vi "prepareToAck.vi"(8 "error in (no error)":errorcluster, 9 "cmdStatus":string(combo)="ack", 10 "cmd":string, 11 "TcpServer in":refnum<class "TcpServer.lvclass">) -> (0 "error out":errorcluster, 2 "JSON string":string, 3 "TcpServer out":refnum<class "TcpServer.lvclass">)   [LabVIEW 2018, in "TcpServer.lvclass"]
doc: "Prepare the command received to do the acknowledgement to the client."
uses:
  TcpServer.lvclass
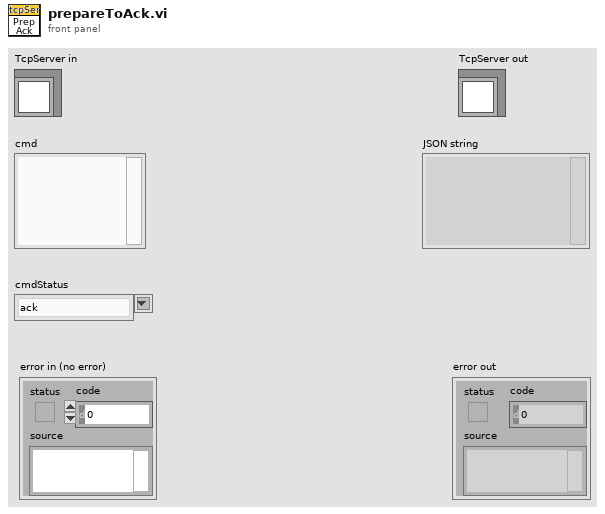
[diagram p1: front panel]
types:
  T1 = cluster{"cmdName":string, "cmdId":i32, "cmdStatus":string}
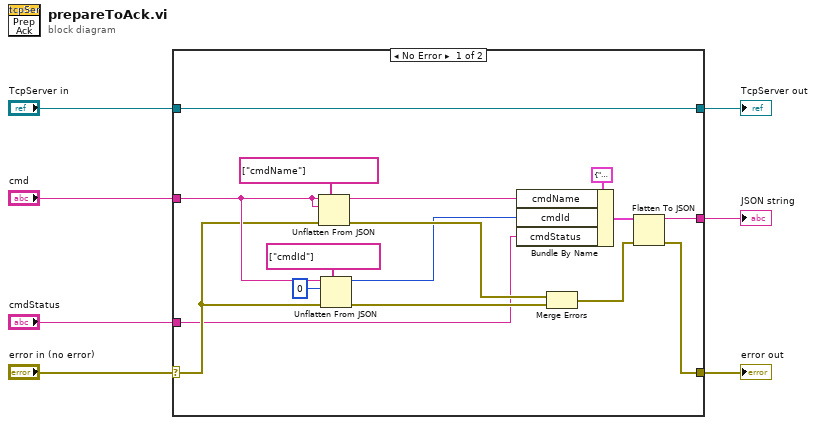
[diagram p0: block diagram]
diagram:
  n1 = case shown="No Error" "error in (no error)" {
    selector: "error in (no error)" -> [w14 w25]
    tunnel: [w10 w25] -> w6
    tunnel: [w23 w24] -> w4
    tunnel: "TcpServer in" -> [w23 w24]
    tunnel: "cmd" -> [w20 _]
    tunnel: [w15 _] -> w2
    tunnel: "cmdStatus" -> [w8 _]
    frame No Error {
      n2 = Unflatten From JSON(path=string[] ["cmdName"], JSON string=w20, type and defaults=w20, error in (no error)=w14) -> (value=w17:string, error out=w13:errorcluster)  [unwired: 3 in]
      n3 = Unflatten From JSON(path=string[] ["cmdId"], JSON string=w20, type and defaults=0, error in (no error)=w14) -> (value=w9:i32, error out=w12:errorcluster)  [unwired: 3 in]
      n4 = Bundle By Name(cluster=T1 {"cmdName"="", "cmdId"=0, "cmdStatus"=""}, "cmdName"=w17, "cmdId"=w9, "cmdStatus"=w8) -> (w16:T1)
      n5 = Merge Errors(w13, w12) -> (w11:errorcluster)
      n6 = Flatten To JSON(anything=w16, error in (no error)=w11) -> (JSON string=w15:string, 11:w10:errorcluster)  [unwired: 1 in]
    }
    frame Error {
    }
  }
  "error out" <- w6
  "TcpServer out" <- w4
  "JSON string" <- w2
